vi "CRYPEAQ IntNoise.vi"(11 "fc":dbl[](array[numeric])) -> (3 "EIN":dbl[](array[numeric]))   [LabVIEW 2013]
panel:
  out "Internal Noise":cluster{"f":dbl[], dbl[]}(graph)
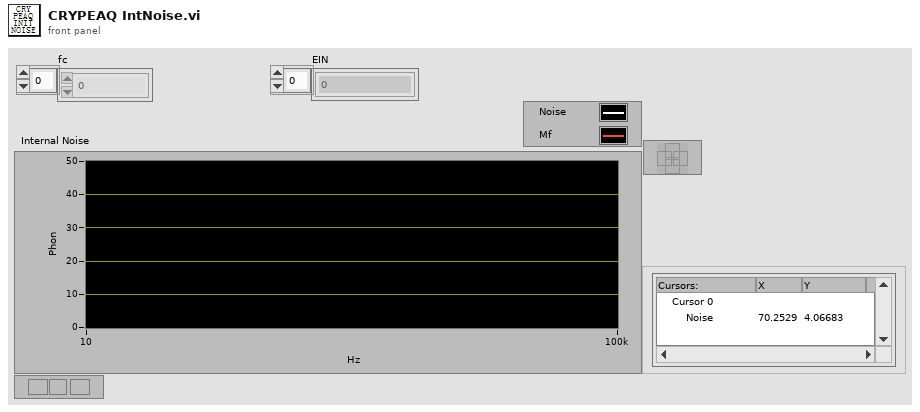
[diagram p1: front panel]
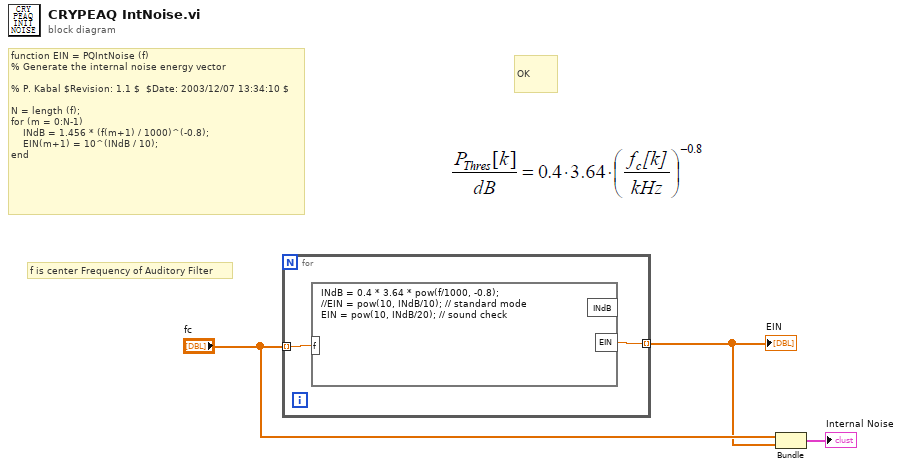
[diagram p0: block diagram]
diagram:
  # "OK"
  # "function EIN = PQIntNoise (f)\n% Generate the internal noise energy vector\n\n% P. Kabal $Revision: 1.1 $  $Date: 2003/12/07 13:34:10 $\n\nN = length (f);\nfor (m = 0:N-1)\n    INdB = 1.456 * (f(m+1) / 1000)^(-0.8);\n    EIN(m+1) = 10^(INdB / 10);\nend"
  # "f is center Frequency of Auditory Filter"
  n1 = for {
    tunnel: [w5] -> w2 mode=indexing
    tunnel: "fc" -> [w4] mode=indexing
    n2 = formula code="INdB = 0.4 * 3.64 * pow(f/1000, -0.8);\n//EIN = pow(10, INdB/10); // standard mode\nEIN = pow(10, INdB/20); // sound check"("f"=w4) -> ("EIN"=w5:dbl)  [unwired: 1 out]
  }
  "EIN" <- w2
  n3 = Bundle("fc"="fc", w2) -> (→"Internal Noise":cluster{"fc":dbl[], dbl[]})  [unwired: 1 in]
